vi "Check for Fresh Message.vi"(8 "error in":errorcluster, 11 "Network Command Processor in":refnum<class "Network Command Processor.lvclass">) -> (0 "error out":errorcluster, 1 "Enqueuer":refnum<class "Message Enqueuer.lvclass">, 2 "Enqueuer not Valid":bool, 3 "Network Command Processor out":refnum<class "Network Command Processor.lvclass">)   [LabVIEW 2014, in "Network Command Processor.lvclass"]
doc: "This method is a dynamic method that \n1) checks for a good connection to the shared variable. If it is not present, then it attempts to connect If a connection is not available, then this VI will do nothing.\n2) Check the state of the enqueuer. If the state is no good, return with this indication and do nothing.\n2) If the connection is good, check to see if the current shared variable state has changed.\n3) If the state has changed, pump the message into the appropriate enqueuer."
uses:
  Network Command Processor.lvclass
  <vilib>/ActorFramework/Message Enqueuer/Message Enqueuer.lvclass
  Network Command Processor.lvclass/Network Command Processor.ctl
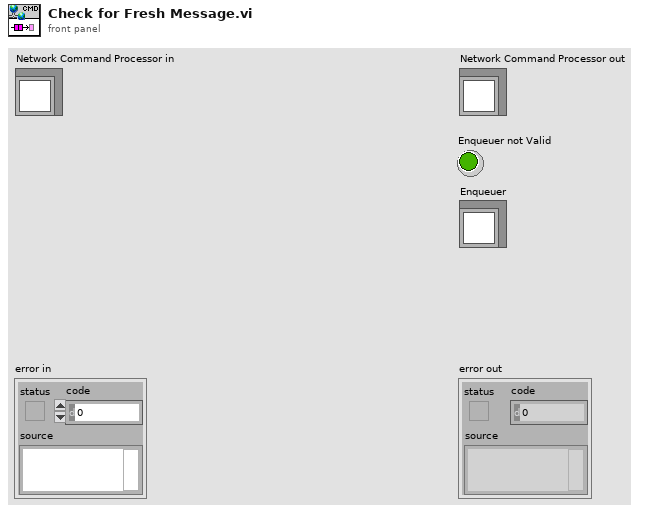
[diagram p1: front panel]
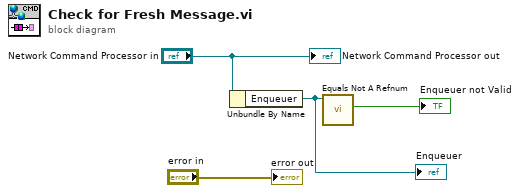
[diagram p0: block diagram]
diagram:
  n1 = Unbundle By Name("Network Command Processor in") -> ("Enqueuer"=w3:refnum<class "Message Enqueuer.lvclass">)
  "Enqueuer" <- w3
  n2 = call <vilib>:"Equals Not A Refnum.vi"("Message Enqueuer"=w3) -> ("Not a refnum?"=→"Enqueuer not Valid":bool)  [unwired: 10 in]
  "error out" <- "error in"
  "Network Command Processor out" <- "Network Command Processor in"
